vi "Add.vi"(7 "LabVIEW Web Service Request":refnum<class "Web Request.lvclass">, 10 "b":dbl format="%#_13g", 11 "a":dbl format="%#_13g") -> (2 "value":string, 3 "c":dbl format="%#_13g")   [LabVIEW 2017]
uses:
  <vilib>/wsapi/Web Request.lvclass
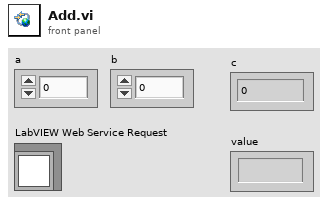
[diagram p1: front panel]
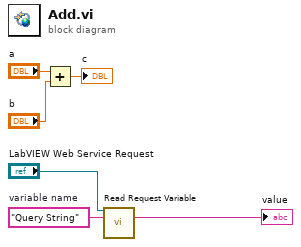
[diagram p0: block diagram]
diagram:
  w1 = "Query String"  # variable name
  n1 = Add(x="a", y="b") -> (x+y=→"c":dbl)
  n2 = call <vilib>:"Read Request Variable.vi"("LabVIEW Web Service Request"="LabVIEW Web Service Request", "variable name"=w1) -> ("value"=→"value":string)  [unwired: 11 in, 2 out]
